vi "dfd_FXP PtByPt Direct FIR.vi"(6 "state in":i64[](array[numeric]), 7 "FXPOPs":T5[](array[typedef]) {"source" items=["Coef a/k"=0, "Coef b/v"=7, "Input"=1, "Output"=2, "Multiplicand"=3, "Product"=4, "Sum"=5, "Delay"=6, "Gain"=8]}, 8 "filtering statistics in":T4(array[cluster]) {"statistics information"."min value" format="%.2f"; "statistics information"."max value" format="%.2f"; "Quantizer Source" items=["Coefficients a/k"=0, "Coefficients b/v"=7, "Input"=1, "Output"=2, "Multiplicand"=3, "Product"=4, "Sum"=5, "Delay"=6]}, 10 "coef b":T1, 11 "x":T7={"value"=0, "wl"=0, "iwl"=0, "Signed"=TRUE} {"value" format="%.0x"}) -> (0 "filtering statistics out":T4(array[cluster]) {"statistics information"."min value" format="%.2f"; "statistics information"."max value" format="%.2f"; "Quantizer Source" items=["Coefficients a/k"=0, "Coefficients b/v"=7, "Input"=1, "Output"=2, "Multiplicand"=3, "Product"=4, "Sum"=5, "Delay"=6]}, 3 "filtered x":T7={"value"=0, "wl"=0, "iwl"=0, "Signed"=TRUE} {"value" format="%.0x"}, 4 "state out":i64[](array[numeric]))   [LabVIEW 2017, in "NI_DigFilter_FXP.lvlib"]
uses:
  <vilib>/addons/Digital Filter Design/NI_DigFilter_FXP.lvlib
  <vilib>/addons/Digital Filter Design/_Objects.llb/dfd_DFXP Data Type (scaler).ctl
  <vilib>/addons/Digital Filter Design/_Objects.llb/dfd_DFXP Operation Parameter.ctl
  <vilib>/addons/Digital Filter Design/_Objects.llb/dfd_Internal Quantization Srcs.ctl
  <vilib>/addons/Digital Filter Design/_Objects.llb/dfd_DFXP Data Type (vector).ctl
  <vilib>/addons/Digital Filter Design/_Objects.llb/DFD Quantization Sources.ctl
  <vilib>/addons/Digital Filter Design/_Objects.llb/DFD FXP Statistics Data.ctl
  <vilib>/addons/Digital Filter Design/NI_DigFilterLicensed.lvlib
panel:
  in  "state":T1
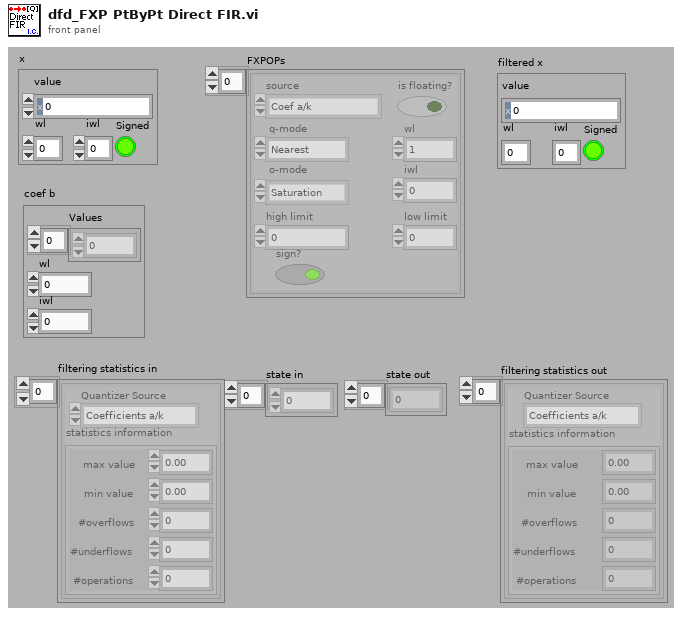
[diagram p1: front panel]
types:
  T1 = typedef "dfd_DFXP Data Type (vector).ctl" = cluster{"Values":i64[], "wl":i16, "iwl":i16}
  T2 = typedef "NI_DigFilterLicensed.lvlib/DFD Quantization Sources.ctl" = u16
  T3 = typedef "NI_DigFilterLicensed.lvlib/DFD FXP Statistics Data.ctl" = cluster{"max value":ext, "min value":ext, "#overflows":i32, "#underflows":i32, "#operations":i32}
  T4 = cluster{"Quantizer Source":T2, "statistics information":T3}[]
  T5 = typedef "dfd_DFXP Operation Parameter.ctl" = cluster{"source":T6, "is floating?":bool, "o-mode":enum16{"Saturation", "Wrap"}, "q-mode":enum16{"Nearest", "Truncation"}, "wl":i16, "high limit":i64, "low limit":i64, "iwl":i16, "sign?":bool}
  T6 = typedef "NI_DigFilterLicensed.lvlib/dfd_Internal Quantization Srcs.ctl" = u16
  T7 = typedef "dfd_DFXP Data Type (scaler).ctl" = cluster{"value":i64, "wl":i16, "iwl":i16, "Signed":bool}
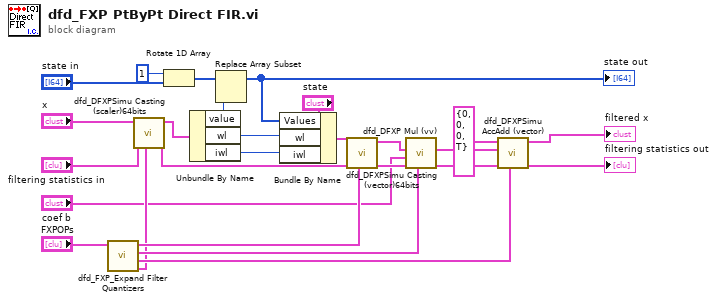
[diagram p0: block diagram]
diagram:
  n1 = call <vilib>:"dfd_FXP_Expand Filter Quantizers.vi"("FXPOPs"="FXPOPs") -> ("Delay"=w11:T5, "Sum"=w12:T5, "Product"=w13:T5, "Multiplicand"=w14:T5)  [unwired: 7 out]
  n2 = call <vilib>:"dfd_DFXPSimu Casting (scaler)64bits.vi"("op params"=w11, "filtering statistics in"="filtering statistics in", "Value in"="x") -> ("filtering statistics out"=w17:T4, "Value out"=w8:T7)  [unwired: 1 in, 6 out]
  n3 = Rotate 1D Array(1:"state in", 2:1 ("n")) -> (0:w18:i64[])
  n4 = Unbundle By Name(w8) -> ("value"=w9:i64, "wl"=w6:i16, "iwl"=w5:i16)
  n5 = Replace Array Subset(array=w18, new element=w9) -> (w20:i64[])  [unwired: 1 in]
  "state out" <- w20
  n6 = Bundle By Name(cluster="state", "Values"=w20, "wl"=w6, "iwl"=w5) -> (w4:T1)
  n7 = call <vilib>:"dfd_DFXPSimu Casting (vector)64bits.vi"("op params"=w14, "filtering statistics in"=w17, "Value in"=w4) -> ("filtering statistics out"=w16:T4, "Value out"=w2:T1)  [unwired: 1 in, 6 out]
  n8 = call <vilib>:"dfd_DFXP Mul (vv).vi"("op params"=w13, "filtering statistics in"=w16, "Value in 2"="coef b", "Value in"=w2) -> ("filtering statistics out"=w15:T4, "Value out"=w1:T1)  [unwired: 6 out]
  n9 = call <vilib>:"dfd_DFXPSimu AccAdd (vector).vi"("op params"=w12, "filtering statistics in"=w15, "addends"=w1, "acc in"=T7 {"value"=0, "wl"=0, "iwl"=0, "Signed"=TRUE}) -> ("filtering statistics out"=→"filtering statistics out":T4, "acc out"=→"filtered x":T7)  [unwired: 1 in, 5 out]
